vi "Move Labels Sub.vi"(6 "Variant in":variant, 7 "Shift Pressed?":bool, 8 "error in (no error)":errorcluster, 10 "QD Combo Box Ref":refnum<vi>, 11 "QD Launch VI Ref":refnum<vi>) -> (0 "error out":errorcluster, 4 "Variant out":variant)   [LabVIEW 2017]
doc: "Repositions the visible labels or captions of top-level front panel and block diagram objects to be consistent with the \"Default label position\" settings in Tools > Options. If [Shift] is also pressed, then all objects, including nested objects, are modified. If this shortcut is activated from the front panel, then controls and indicators are modified. If it is activated from the block diagram, then control and indicator terminals are modified. If panel or diagram objects were already selected when this shortcut is activated, only the selected objects that have visible labels or captions are modified.\n\nThe text justification of the modified labels and captions is also modified to be consistent with the new label or caption position."
uses:
  <vilib>/Utility/traverseref.llb/VI Scripting - Traverse.lvlib
  <vilib>/Utility/traverseref.llb/TRef TravTarget.ctl
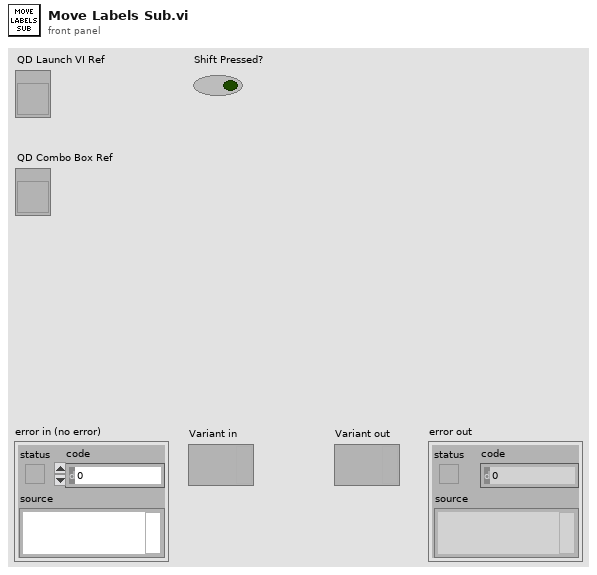
[diagram p1: front panel]
types:
  T1 = typedef "TRef TravTarget.ctl" = enum16{"FP", "BD", "Other"}
  T2 = typedef "LVRectTypeDef.ctl" = cluster{"Left":i16, "Top":i16, "Right":i16, "Bottom":i16}
  T3 = cluster{"MasterRect":T2, "Label":refnum<vi>, "f":i32}
  T4 = enum32{"None", "Size to Fit", "Arrange Horizontally", "Arrange Vertically"}
  T5 = cluster{"Bounds Rect":T2, "Label":refnum<vi>, "f":i32}
  T6 = cluster{"Bounds Rect":T2, "Label":refnum<vi>, "right-top":i32}
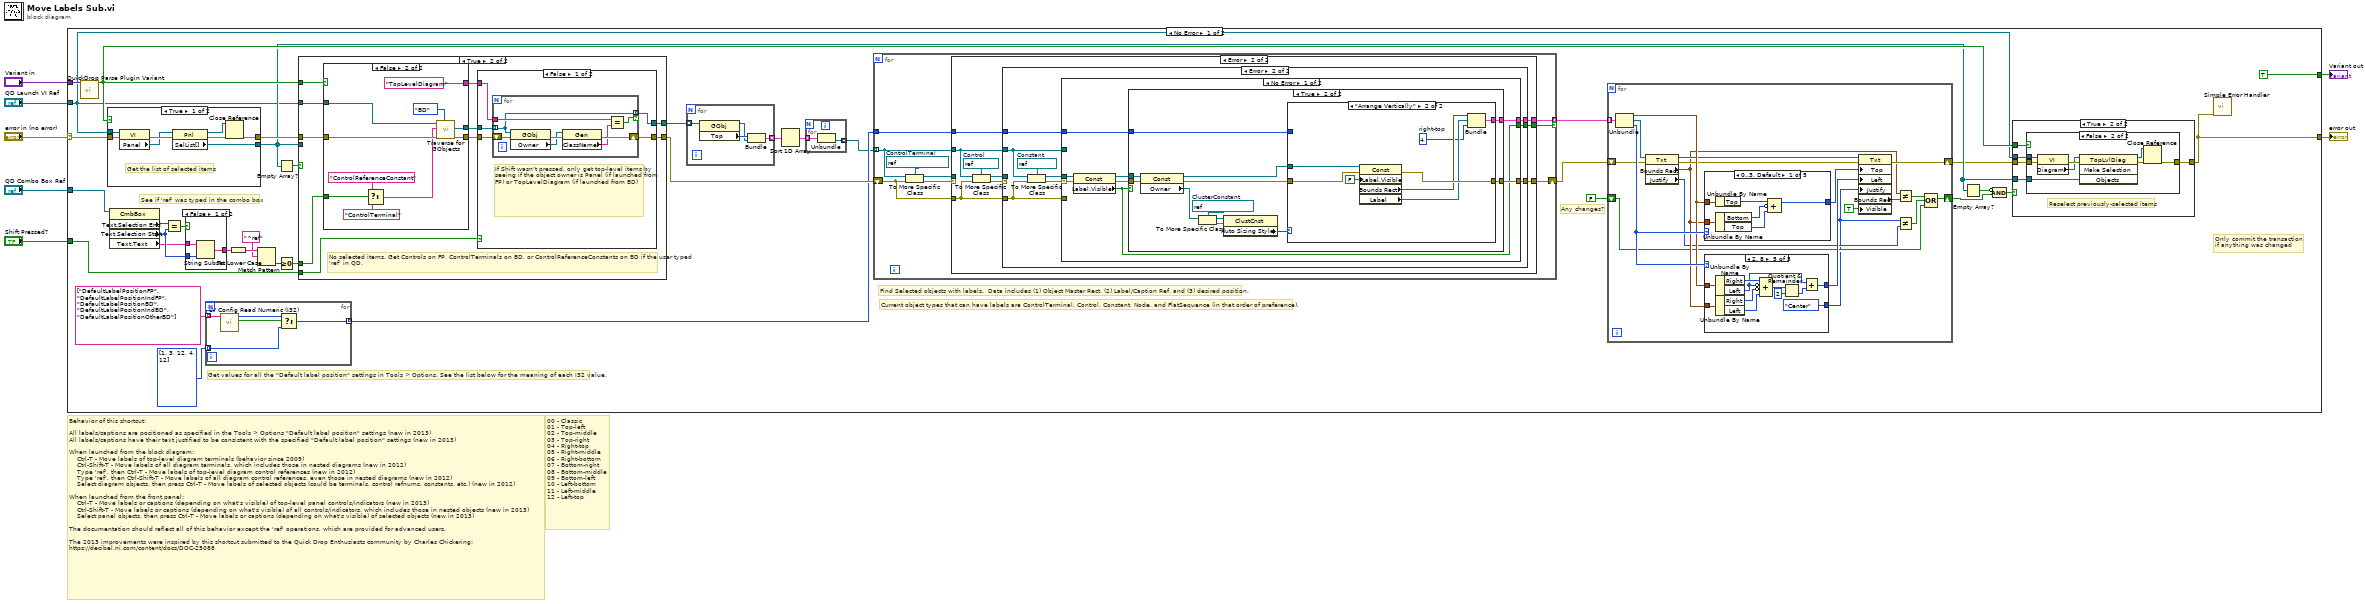
[diagram p0: block diagram]
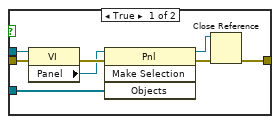
[diagram p3: hidden frame]
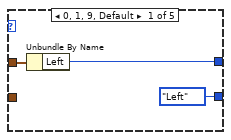
[diagram p4: hidden frame]
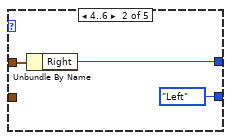
[diagram p5: hidden frame]
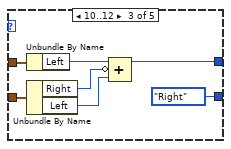
[diagram p6: hidden frame]
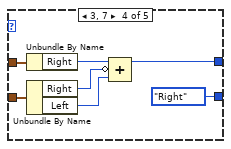
[diagram p7: hidden frame]
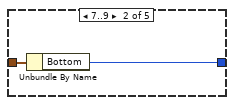
[diagram p8: hidden frame]
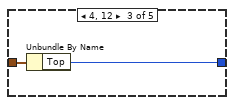
[diagram p9: hidden frame]
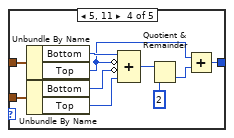
[diagram p10: hidden frame]
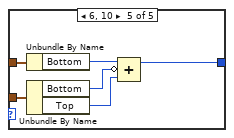
[diagram p11: hidden frame]
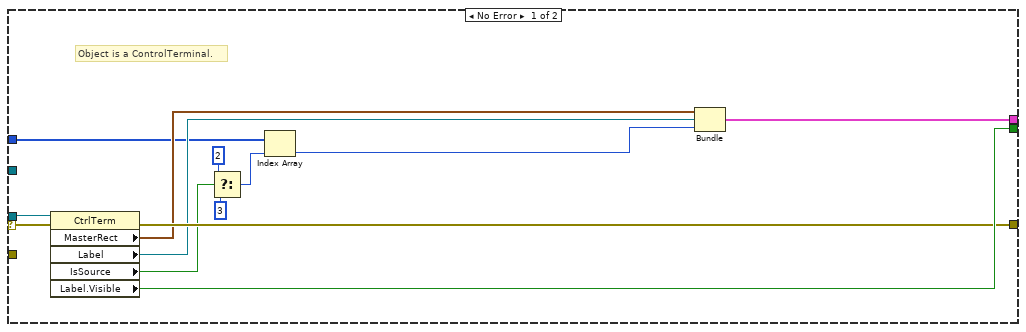
[diagram p12: hidden frame]
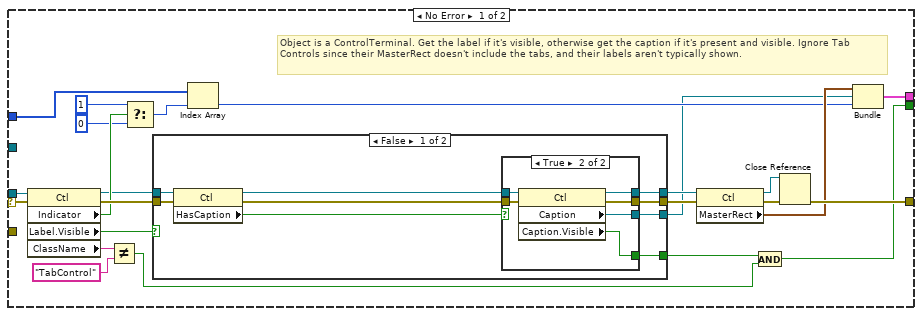
[diagram p13: hidden frame]
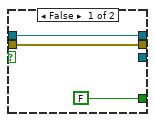
[diagram p14: hidden frame]
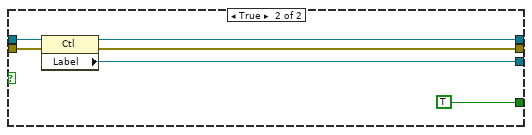
[diagram p15: hidden frame]
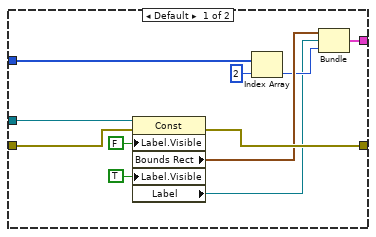
[diagram p17: hidden frame]
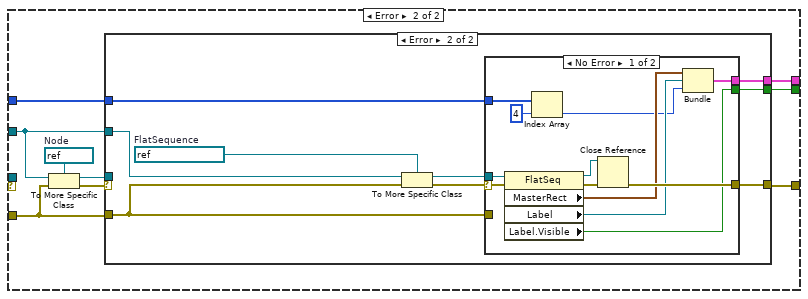
[diagram p18: hidden frame]
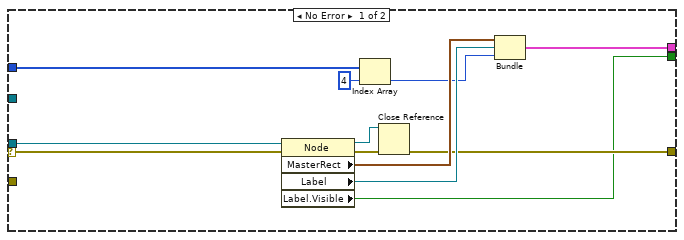
[diagram p19: hidden frame]
diagram:
  # "00 - Classic\n01 - Top-left\n02 - Top-middle\n03 - Top-right\n04 - Right-top\n05 - Right-middle\n06 - Right-bottom\n07 - Bottom-right\n08 - Bottom-middle\n09 - Bottom-left\n10 - Left-bottom\n11 - Left-middle\n12 - Left-top"
  # "Behavior of this shortcut:\n\nAll labels/captions are positioned as specified in the Tools > Options \"Default label position\" settings (new in 2013)\nAll labels/captions have their text justified to be consistent with the specified \"Default label position\" settings (new in 2013) \n\nWhen launched from the block diagram:\n    Ctrl-T - Move labels of top-level diagram terminals (behavior since 2009)\n    Ctrl-Shift-T - Move labels of all diagram terminals, which includes those in nested diagrams (new in 2012)\n    Type 'ref', then Ctrl-T - Move labels of top-level diagram control references (new in 2012)\n    Type 'ref', then Ctrl-Shift-T - Move labels of all diagram control references, even those in nested diagrams (new in 2012)\n    Select diagram objects, then press Ctrl-T - Move labels of selected objects (could be terminals, control refnums, constants, etc.) (new in 2012)\n\nWhen launched from the front panel:\n    Ctrl-T - Move labels or captions (depending on what's visible) of top-level panel controls/indicators (new in 2013)\n    Ctrl-Shift-T - Move labels or captions (depending on what's visible) of all controls/indicators, which includes those in nested objects (new in 2013)\n    Select panel objects, then press Ctrl-T - Move labels or captions (depending on what's visible) of selected objects (new in 2013)\n\nThe documentation should reflect all of this behavior except the 'ref' operations, which are provided for advanced users.\n\nThe 2013 improvements were inspired by this shortcut submitted to the Quick Drop Enthusiasts community by Charles Chickering:\nhttps://decibel.ni.com/content/docs/DOC-25088"
  n1 = case shown="No Error" "error in (no error)" {
    selector: "error in (no error)" -> [w42 w387]
    tunnel: [w16 w387] -> w6
    tunnel: "Shift Pressed?" -> [w28 _]
    tunnel: "QD Launch VI Ref" -> [w13 _]
    tunnel: "QD Combo Box Ref" -> [w33 _]
    tunnel: "Variant in" -> [w41 _]
    tunnel: [TRUE _] -> w1
    frame No Error {
      # "Get values for all the \"Default label position\" settings in Tools > Options. See the list below for the meaning of each I32 value."
      # "Current object types that can have labels are ControlTerminal, Control, Constant, Node, and FlatSequence (in that order of preference)."
      # "Find Selected objects with labels.  Data includes (1) Object Master Rect, (2) Label/Caption Ref, and (3) desired position."
      # "See if 'ref' was typed in the combo box"
      # "Any changes?"
      # "Only commit the transaction\nif anything was changed"
      n2 = call <vilib>:"QuickDrop Parse Plugin Variant.vi"("QDKS Variant in"=w41) -> ("QD Launch VI Panel?"=w24:bool)  [unwired: 12 in, 2 out]
      n3 = case shown="True" w24 {
        tunnel: w13 -> [w374 w382]
        tunnel: w42 -> [w373 w381]
        tunnel: [w372 w380] -> w30
        tunnel: [w371 w379] -> w22
        frame True {
          # "Get the list of selected items"
          n4 = property class="VI"(reference=w374, error in=w373) -> (error out=w378:errorcluster, "Panel"=w377:refnum<vi>)  [unwired: 1 out]
          n5 = property class="Pnl"(reference=w377, error in=w378) -> (reference out=w375:refnum<vi>, error out=w376:errorcluster, "SelList[]"=w371:refnum<vi>[])
          n6 = Close Reference(reference=w375, error in (no error)=w376) -> (error out=w372:errorcluster)
        }
        frame False {
          # "Get the list of selected items"
          n7 = property class="VI"(reference=w382, error in=w381) -> (error out=w386:errorcluster, "Diagram"=w385:refnum<vi>)  [unwired: 1 out]
          n8 = property class="TopLvlDiag"(reference=w385, error in=w386) -> (reference out=w383:refnum<vi>, error out=w384:errorcluster, "SelList[]"=w379:refnum<vi>[])
          n9 = Close Reference(reference=w383, error in (no error)=w384) -> (error out=w380:errorcluster)
        }
      }
      n10 = property on="Property Node" class="CmbBox"(reference=w33) -> ("Text.Selection End"=w40:u32, "Text.Selection Start"=w38:u32, "Text.Text"=w37:string)  [unwired: 1 in, 2 out]
      n11 = Equal?(x=w40, y=w38) -> (x = y?=w39:bool)
      n12 = case shown="False" w39 {
        tunnel: [w369 w370] -> w36
        tunnel: w38 -> [w368 _]
        tunnel: w37 -> [w367 w370]
        frame False {
          n13 = String Subset(string=w367, length (rest)=w368) -> (substring=w369:string)  [unwired: 1 out]
        }
        frame True {
        }
      }
      n14 = for {
        tunnel: string[] ["DefaultLabelPositionFP", "DefaultLabelPositionIndFP", "DefaultLabelPositionBD", "DefaultLabelPositionIndBD", "DefaultLabelPositionOtherBD"] -> [w53] mode=indexing
        tunnel: [w50] -> w12 mode=indexing
        tunnel: i32[] [1, 3, 12, 4, 12] -> [w49] mode=indexing
        n15 = call <resource>:"LV Config Read Numeric (I32).vi"("key"=w53) -> ("found?"=w52:bool, "value"=w51:i32)  [unwired: 4 in, 1 out]
        n16 = Select(t=w51, s=w52, f=w49) -> (s? t:f=w50:i32)
      }
      n17 = To Lower Case(string=w36) -> (all lower case string=w35:string)
      n18 = Match Pattern(string=w35, regular expression="^ref") -> (offset past match=w32:i32)  [unwired: 1 in, 3 out]
      n19 = Empty Array?(array=w22) -> (empty?=w31:bool)
      n20 = Greater Or Equal To 0?(x=w32) -> (x >= 0?=w29:bool)
      n21 = case shown="True" w31 {
        tunnel: w22 -> [w324 _]
        tunnel: w30 -> [w323 w333]
        tunnel: [w324 w326] -> w11
        tunnel: w24 -> [_ w334]
        tunnel: w29 -> [_ w331]
        tunnel: w13 -> [_ w332]
        tunnel: w28 -> [_ w328]
        tunnel: [w323 w327] -> w14
        frame False {
          # "There were selected items. Only operate on those."
        }
        frame True {
          # "No selected items. Get Controls on FP, ControlTerminals on BD, or ControlReferenceConstants on BD if the user typed 'ref' in QD."
          n22 = case shown="False" w334 {
            tunnel: w333 -> [w356 w366]
            tunnel: w332 -> [w355 w365]
            tunnel: [w352 w363] -> w330
            tunnel: [w351 w362] -> w329
            tunnel: ["Panel" "TopLevelDiagram"] -> w325
            tunnel: w331 -> [_ w360]
            frame True {
              n23 = call <vilib>:"Traverse for GObjects.vi"("Traverse Target"=TRef_TravTarget."FP", "error in (no error)"=w356, "Class Name"="Control", "VI Refnum"=w355) -> ("error out"=w352:errorcluster, "References"=w351:refnum<vi>[])  [unwired: 4 in, 2 out]
            }
            frame False {
              n24 = Select(t="ControlReferenceConstant", s=w360, f="ControlTerminal") -> (s? t:f=w359:string)
              n25 = call <vilib>:"Traverse for GObjects.vi"("Traverse Target"=TRef_TravTarget."BD", "error in (no error)"=w366, "Class Name"=w359, "VI Refnum"=w365) -> ("error out"=w363:errorcluster, "References"=w362:refnum<vi>[])  [unwired: 4 in, 2 out]
            }
          }
          n26 = case shown="False" w328 {
            tunnel: w330 -> [w339 w349]
            tunnel: w329 -> [w338 w348]
            tunnel: [w336 w349] -> w327
            tunnel: [w335 w348] -> w326
            tunnel: w325 -> [w337 _]
            frame False {
              # "If Shift wasn't pressed, only get top-level items by seeing if the object owner is Panel (if launched from FP) or TopLevelDiagram (if launched from BD)"
              n27 = for {
                shift-right: [w344] -> w336
                shift-left: w339 -> [w347]
                tunnel: w338 -> [w341] mode=indexing
                tunnel: w337 -> [w342]
                tunnel: [w341] -> w335 mode=indexing if=w340
                n28 = property class="GObj"(reference=w341, error in=w347) -> (error out=w346:errorcluster, "Owner"=w345:refnum<vi>)  [unwired: 1 out]
                n29 = property class="Gen"(reference=w345, error in=w346) -> (error out=w344:errorcluster, "ClassName"=w343:string)  [unwired: 1 out]
                n30 = Equal?(x=w342, y=w343) -> (x = y?=w340:bool)
              }
            }
            frame True {
            }
          }
        }
      }
      n31 = for {
        tunnel: w11 -> [w48] mode=indexing
        tunnel: [w45] -> w10 mode=indexing
        n32 = property class="GObj"(reference=w48) -> (reference out=w46:refnum<vi>, "Top"=w47:i32)  [unwired: 1 in, 1 out]
        n33 = Bundle("Top"=w47, w46) -> (w45:cluster{"Top":i32, refnum<vi>})  [unwired: 1 in]
      }
      n34 = Sort 1D Array(array=w10) -> (sorted array=w9:cluster{"Top":i32, refnum<vi>}[])
      n35 = for {
        tunnel: w9 -> [w44] mode=indexing
        tunnel: [w43] -> w8 mode=indexing
        n36 = Unbundle(w44) -> (w43:refnum<vi>)  [unwired: 1 out]
      }
      n37 = for {
        shift-right: [w160] -> w15
        shift-left: w14 -> [w152]
        tunnel: w8 -> [w158] mode=indexing
        tunnel: [w159] -> w27 mode=indexing if=w154
        tunnel: w12 -> [w153]
        w155 = refnum<vi> refnum  # ControlTerminal
        n38 = To More Specific Class(target class=w155, reference=w158, error in=w152) -> (specific class reference=w156:refnum<vi>, error out=w157:errorcluster)
        n39 = case shown="Error" w157 {
          selector: w157 -> [w172 _]
          tunnel: [w170 w179] -> w160
          tunnel: w158 -> [_ w178]
          tunnel: [w167 w177] -> w159
          tunnel: w156 -> [w173 _]
          tunnel: [w171 w175] -> w154
          tunnel: w153 -> [w166 w176]
          tunnel: w152 -> [_ w174]
          frame No Error {
            # "Object is a ControlTerminal."
            n40 = property class="CtrlTerm"(reference=w173, error in=w172) -> (error out=w170:errorcluster, "MasterRect"=w169:T2, "Label"=w168:refnum<vi>, "IsSource"=w165:bool, "Label.Visible"=w171:bool)  [unwired: 1 out]
            n41 = Select(t=2, s=w165, f=3) -> (s? t:f=w162:i32)
            n42 = Index Array(array=w166, index=w162) -> (element=w161:i32)
            n43 = Bundle("MasterRect"=w169, "Label"=w168, "f"=w161) -> (w167:T3)  [unwired: 1 in]
          }
          frame Error {
            w182 = refnum<vi> refnum  # Control
            n44 = To More Specific Class(target class=w182, reference=w178, error in=w174) -> (specific class reference=w181:refnum<vi>, error out=w180:errorcluster)
            n45 = case shown="Error" w180 {
              selector: w180 -> [w206 _]
              tunnel: w181 -> [w199 _]
              tunnel: [w203 w235] -> w179
              tunnel: w174 -> [_ w236]
              tunnel: w178 -> [_ w234]
              tunnel: [w201 w233] -> w177
              tunnel: w176 -> [w187 w231]
              tunnel: [w184 w232] -> w175
              frame No Error {
                # "Object is a ControlTerminal. Get the label if it's visible, otherwise get the caption if it's present and visible. Ignore Tab Controls since their MasterRect doesn't include the tabs, and their labels aren't typically shown."
                n46 = property class="Ctl"(reference=w199, error in=w206) -> (reference out=w192:refnum<vi>, error out=w200:errorcluster, "Indicator"=w198:bool, "Label.Visible"=w190:bool, "ClassName"=w186:string)
                n47 = Not Equal?(x=w186, y="TabControl") -> (x != y?=w183:bool)
                n48 = Select(t=1, s=w198, f=0) -> (s? t:f=w195:i32)
                n49 = case shown="False" w190 {
                  tunnel: w200 -> [w215 w230]
                  tunnel: [w212 w227] -> w193
                  tunnel: w192 -> [w213 w229]
                  tunnel: [w210 w228] -> w191
                  tunnel: [w208 w226] -> w189
                  tunnel: [w207 TRUE] -> w188
                  frame False {
                    n50 = property class="Ctl"(reference=w213, error in=w215) -> (reference out=w211:refnum<vi>, error out=w214:errorcluster, "HasCaption"=w209:bool)
                    n51 = case shown="True" w209 {
                      tunnel: w214 -> [w217 w224]
                      tunnel: [w217 w223] -> w212
                      tunnel: w211 -> [w218 w222]
                      tunnel: [w218 w221] -> w210
                      tunnel: [_ w220] -> w208
                      tunnel: [FALSE w219] -> w207
                      frame False {
                      }
                      frame True {
                        n52 = property class="Ctl"(reference=w222, error in=w224) -> (reference out=w221:refnum<vi>, error out=w223:errorcluster, "Caption"=w220:refnum<vi>, "Caption.Visible"=w219:bool)
                      }
                    }
                  }
                  frame True {
                    n53 = property class="Ctl"(reference=w229, error in=w230) -> (reference out=w228:refnum<vi>, error out=w227:errorcluster, "Label"=w226:refnum<vi>)
                  }
                }
                n54 = Index Array(array=w187, index=w195) -> (element=w194:i32)
                n55 = property class="Ctl"(reference=w191, error in=w193) -> (reference out=w204:refnum<vi>, error out=w205:errorcluster, "MasterRect"=w202:T2)
                n56 = And(x=w188, y=w183) -> (x .and. y?=w184:bool)
                n57 = Close Reference(reference=w204, error in (no error)=w205) -> (error out=w203:errorcluster)
                n58 = Bundle("MasterRect"=w202, "Label"=w189, "f"=w194) -> (w201:T3)  [unwired: 1 in]
              }
              frame Error {
                w239 = refnum<vi> refnum  # Constant
                n59 = To More Specific Class(target class=w239, reference=w234, error in=w236) -> (specific class reference=w237:refnum<vi>, error out=w238:errorcluster)
                n60 = case shown="No Error" w238 {
                  selector: w238 -> [w247 _]
                  tunnel: w236 -> [_ w284]
                  tunnel: w237 -> [w242 _]
                  tunnel: [w246 w285] -> w235
                  tunnel: w234 -> [_ w283]
                  tunnel: [w245 w282] -> w233
                  tunnel: [w240 w281] -> w232
                  tunnel: w231 -> [w244 w280]
                  frame No Error {
                    n61 = property class="Const"(reference=w242, error in=w247) -> (reference out=w241:refnum<vi>, error out=w243:errorcluster, "Label.Visible"=w240:bool)
                    n62 = case shown="True" w240 {
                      tunnel: [w248 w260] -> w246
                      tunnel: [_ w259] -> w245
                      tunnel: w244 -> [_ w258]
                      tunnel: w243 -> [w248 w257]
                      tunnel: w241 -> [_ w255]
                      frame False {
                      }
                      frame True {
                        w252 = refnum<vi> refnum  # ClusterConstant
                        n63 = property class="Const"(reference=w255, error in=w257) -> (reference out=w254:refnum<vi>, error out=w256:errorcluster, "Owner"=w253:refnum<vi>)
                        n64 = To More Specific Class(target class=w252, reference=w253) -> (specific class reference=w250:refnum<vi>, error out=w251:errorcluster)  [unwired: 1 in]
                        n65 = property class="ClustCnst"(reference=w250, error in=w251) -> ("Auto Sizing Style"=w249:T4)  [unwired: 2 out]
                        n66 = case shown="\"Arrange Vertically\"" w249 {
                          tunnel: [w271 w279] -> w260
                          tunnel: [w269 w277] -> w259
                          tunnel: w258 -> [w268 _]
                          tunnel: w256 -> [w262 w274]
                          tunnel: w254 -> [w261 w273]
                          frame Default {
                            n67 = property class="Const"(reference=w261, error in=w262, "Label.Visible"=FALSE, "Label.Visible"=TRUE) -> (error out=w271:errorcluster, "Bounds Rect"=w270:T2, "Label"=w265:refnum<vi>)  [unwired: 1 out]
                            n68 = Index Array(array=w268, index=2) -> (element=w266:i32)
                            n69 = Bundle("Bounds Rect"=w270, "Label"=w265, "f"=w266) -> (w269:T5)  [unwired: 1 in]
                          }
                          frame "Arrange Vertically" {
                            w272 = 4  # right-top
                            n70 = property class="Const"(reference=w273, error in=w274, "Label.Visible"=FALSE) -> (error out=w279:errorcluster, "Bounds Rect"=w278:T2, "Label"=w276:refnum<vi>)  [unwired: 1 out]
                            n71 = Bundle("Bounds Rect"=w278, "Label"=w276, "right-top"=w272) -> (w277:T6)  [unwired: 1 in]
                          }
                        }
                      }
                    }
                  }
                  frame Error {
                    w288 = refnum<vi> refnum  # Node
                    n72 = To More Specific Class(target class=w288, reference=w283, error in=w284) -> (specific class reference=w286:refnum<vi>, error out=w287:errorcluster)
                    n73 = case shown="Error" w287 {
                      selector: w287 -> [w300 _]
                      tunnel: w286 -> [w298 _]
                      tunnel: [w295 w304] -> w285
                      tunnel: w284 -> [_ w305]
                      tunnel: w283 -> [_ w308]
                      tunnel: [w293 w303] -> w282
                      tunnel: [w292 w301] -> w281
                      tunnel: w280 -> [w291 w302]
                      frame No Error {
                        n74 = property class="Node"(reference=w298, error in=w300) -> (reference out=w294:refnum<vi>, error out=w299:errorcluster, "MasterRect"=w297:T2, "Label"=w296:refnum<vi>, "Label.Visible"=w292:bool)
                        n75 = Index Array(array=w291, index=4) -> (element=w289:i32)
                        n76 = Close Reference(reference=w294, error in (no error)=w299) -> (error out=w295:errorcluster)
                        n77 = Bundle("MasterRect"=w297, "Label"=w296, "f"=w289) -> (w293:T3)  [unwired: 1 in]
                      }
                      frame Error {
                        w309 = refnum<vi> refnum  # FlatSequence
                        n78 = To More Specific Class(target class=w309, reference=w308, error in=w305) -> (specific class reference=w306:refnum<vi>, error out=w307:errorcluster)
                        n79 = case shown="No Error" w307 {
                          selector: w307 -> [w321 _]
                          tunnel: w306 -> [w320 _]
                          tunnel: w305 -> [_ w322]
                          tunnel: [w317 w322] -> w304
                          tunnel: [w314 _] -> w303
                          tunnel: w302 -> [w313 _]
                          tunnel: [w310 _] -> w301
                          frame No Error {
                            n80 = property class="FlatSeq"(reference=w320, error in=w321) -> (reference out=w318:refnum<vi>, error out=w319:errorcluster, "MasterRect"=w316:T2, "Label"=w315:refnum<vi>, "Label.Visible"=w310:bool)
                            n81 = Index Array(array=w313, index=4) -> (element=w311:i32)
                            n82 = Close Reference(reference=w318, error in (no error)=w319) -> (error out=w317:errorcluster)
                            n83 = Bundle("MasterRect"=w316, "Label"=w315, "f"=w311) -> (w314:T3)  [unwired: 1 in]
                          }
                          frame Error {
                          }
                        }
                      }
                    }
                  }
                }
              }
            }
          }
        }
      }
      n84 = for {
        tunnel: w27 -> [w94] mode=indexing
        shift-right: [w91] -> w20
        shift-left: w15 -> [w89]
        shift-right: [w78] -> w19
        shift-left: FALSE -> [w79]
        n85 = Unbundle(w94) -> ("MasterRect"=w92:T2, "Label"=w90:refnum<vi>, "f"=w93:i32)
        n86 = property class="Txt"(reference=w90, error in=w89) -> (reference out=w88:refnum<vi>, error out=w86:errorcluster, "Bounds Rect"=w84:T2, "Justify"=w81:enum16{"Left", "Center", "Right"})
        n87 = case shown="0..3, Default" w93 {
          tunnel: w92 -> [w131 w133 w135 w145 w151]
          tunnel: w84 -> [w130 _ _ w144 w150]
          tunnel: [w126 w132 w134 w140 w146] -> w87
          frame 0..3, Default {
            n88 = Unbundle By Name(w131) -> ("Top"=w129:i16)
            n89 = Unbundle By Name(w130) -> ("Bottom"=w128:i16, "Top"=w127:i16)
            n90 = Compound Arithmetic op=ADD(w129, invert w128, w127) -> (w126:i16)
          }
          frame 7..9 {
            n91 = Unbundle By Name(w133) -> ("Bottom"=w132:i16)
          }
          frame 4, 12 {
            n92 = Unbundle By Name(w135) -> ("Top"=w134:i16)
          }
          frame 5, 11 {
            n93 = Unbundle By Name(w145) -> ("Bottom"=w139:i16, "Top"=w138:i16)
            n94 = Unbundle By Name(w144) -> ("Bottom"=w143:i16, "Top"=w142:i16)
            n95 = Compound Arithmetic op=ADD(w139, invert w138, invert w143, w142) -> (w137:i16)
            n96 = Quotient & Remainder(x=w137, y=i16 2) -> (floor(x/y)=w141:i16)  [unwired: 1 out]
            n97 = Add(x=w138, y=w141) -> (x+y=w140:i16)
          }
          frame 6, 10 {
            n98 = Unbundle By Name(w151) -> ("Bottom"=w149:i16)
            n99 = Unbundle By Name(w150) -> ("Bottom"=w148:i16, "Top"=w147:i16)
            n100 = Compound Arithmetic op=ADD(w149, invert w148, w147) -> (w146:i16)
          }
        }
        n101 = case shown="2, 8" w93 {
          tunnel: w92 -> [w97 w100 w107 w114 w123]
          tunnel: w84 -> [_ _ w105 w112 w122]
          tunnel: [w96 w99 w102 w109 w119] -> w82
          tunnel: [enum16{"Left", "Center", "Right"}."Left" ("Justification") enum16{"Left", "Center", "Right"}."Left" ("Justification") enum16{"Left", "Center", "Right"}."Right" ("Justification") enum16{"Left", "Center", "Right"}."Right" ("Justification") enum16{"Left", "Center", "Right"}."Center" ("Justification")] -> w77
          frame 0, 1, 9, Default {
            n102 = Unbundle By Name(w97) -> ("Left"=w96:i16)
          }
          frame 4..6 {
            n103 = Unbundle By Name(w100) -> ("Right"=w99:i16)
          }
          frame 10..12 {
            n104 = Unbundle By Name(w107) -> ("Left"=w106:i16)
            n105 = Unbundle By Name(w105) -> ("Right"=w104:i16, "Left"=w103:i16)
            n106 = Compound Arithmetic op=ADD(w106, invert w104, w103) -> (w102:i16)
          }
          frame 3, 7 {
            n107 = Unbundle By Name(w114) -> ("Right"=w113:i16)
            n108 = Unbundle By Name(w112) -> ("Right"=w111:i16, "Left"=w110:i16)
            n109 = Compound Arithmetic op=ADD(w113, invert w111, w110) -> (w109:i16)
          }
          frame 2, 8 {
            n110 = Unbundle By Name(w123) -> ("Right"=w121:i16, "Left"=w118:i16)
            n111 = Unbundle By Name(w122) -> ("Right"=w124:i16, "Left"=w125:i16)
            n112 = Compound Arithmetic op=ADD(w121, invert w118, invert w124, w125) -> (w116:i16)
            n113 = Quotient & Remainder(x=w116, y=i16 2) -> (floor(x/y)=w120:i16)  [unwired: 1 out]
            n114 = Add(x=w118, y=w120) -> (x+y=w119:i16)
          }
        }
        n115 = property class="Txt"(reference=w88, error in=w86, "Top"=w87, "Left"=w82, "Justify"=w77, "Visible"=TRUE) -> (error out=w91:errorcluster, "Bounds Rect"=w85:T2)  [unwired: 1 out]
        n116 = Not Equal?(x=w84, y=w85) -> (x != y?=w83:bool)
        n117 = Not Equal?(x=w77, y=w81) -> (x != y?=w80:bool)
        n118 = Compound Arithmetic op=OR(w83, w80, w79) -> (w78:bool)
      }
      n119 = Empty Array?(array=w22) -> (empty?=w21:bool)
      n120 = Compound Arithmetic op=AND(invert w21, w19) -> (w23:bool)
      n121 = case shown="True" w23 {
        tunnel: w20 -> [w54 w59]
        tunnel: [w54 w58] -> w16
        tunnel: w13 -> [_ w57]
        tunnel: w24 -> [_ w56]
        tunnel: w22 -> [_ w55]
        frame False {
          # "No changes, and/or no selected items originally"
        }
        frame True {
          # "Reselect previously-selected items"
          n122 = case shown="False" w56 {
            tunnel: w57 -> [w63 w71]
            tunnel: w59 -> [w62 w70]
            tunnel: [w61 w69] -> w58
            tunnel: w55 -> [w60 w68]
            frame True {
              n123 = property class="VI"(reference=w63, error in=w62) -> (error out=w67:errorcluster, "Panel"=w66:refnum<vi>)  [unwired: 1 out]
              n124 = invoke class="Pnl" method="Make Selection"(reference=w66, error in=w67, "Objects"=w60) -> (reference out=w64:refnum<vi>, error out=w65:errorcluster)  [unwired: 1 in, 2 out]
              n125 = Close Reference(reference=w64, error in (no error)=w65) -> (error out=w61:errorcluster)
            }
            frame False {
              n126 = property class="VI"(reference=w71, error in=w70) -> (error out=w75:errorcluster, "Diagram"=w74:refnum<vi>)  [unwired: 1 out]
              n127 = invoke class="TopLvlDiag" method="Make Selection"(reference=w74, error in=w75, "Objects"=w68) -> (reference out=w72:refnum<vi>, error out=w73:errorcluster)  [unwired: 1 in, 2 out]
              n128 = Close Reference(reference=w72, error in (no error)=w73) -> (error out=w69:errorcluster)
            }
          }
        }
      }
      n129 = call <vilib>:"Simple Error Handler.vi"("error in (no error)"=w16) -> ()  [unwired: 4 in, 5 out]
    }
    frame Error {
    }
  }
  "error out" <- w6
  "Variant out" <- w1
